vi "PRI.vi"(8 "Stopp":bool, 10 "SLOT":i32=100 min=0 max=999 step=100 format="%03d", 11 "USB":i32) -> ()   [LabVIEW 2020]
doc: "This VI provides a GUI for PRI modules. It implements an abstract module interface, where callers provide the only necessary and sufficient information for callee modules via the datafields USB, SLOT and Stopp. All module intern information are handled hidden by the module. Thereby, a caller must not \"know\" about such internals."
panel:
  out "Zeroed Intens":sgl[](array[numeric]) format="%.1f %%"
  in  "WL_Index":i32(ring) caption="Wavelength" items=["450 nm", "515 nm", "640 nm"]
  out "Wavelengths":i32[](array[numeric]) format="%.0f nm"
  in  "ZeroBtn":bool caption="Boolean"
  in  "Intensity":sgl min=0 max=100 step=1 format="%.1f %%"
  out "OnTime":i32=421 min=1000 max=200000000 step=1000 format="%5d ns"
  out "OffFactLo":i32=421 min=1000 max=200000000 step=1000 format="%5d * On-Time"
  out "OffFactHi":i32=421 min=1000 max=200000000 step=1000 format="%5d * On-Time"
  out "OnTimeLo":i32=421 min=1000 max=200000000 step=1000 format="%5d ns"
  out "OnTimeHi":i32=421 min=1000 max=200000000 step=1000 format="%5d ns"
  out "FreqLo":i32=421 min=1000 max=200000000 step=1000 format="%5d Hz"
  out "FreqHi":i32=421 min=1000 max=200000000 step=1000 format="%5d Hz"
  in  "FreqUnitPrefix":i32(ring) items=["Hz"=0, "kHz"=3, "MHz"=6]
  in  "Gating":enum32{"Timing", "Impedance"}(tab)
  in  "Gate Enabled":bool
  in  "OnTimeUnitPrefix":i32(ring) items=["s"=9, "ms"=6, "µs"=3, "ns"=0]
  in  "OnTimeMant":sgl=384.0 caption="On-Time" min=0 max=1000 step=1 format="%.1f"
  in  "OffFact":i32=255 caption="Off-Time" min=1 max=255 step=1 format="%5d * On-Time"
  in  "Gate Impedance":enum32{"   Low", "   High"}(radio)
  out "Frequency":i32=421 min=1000 max=200000000 step=1000 format="%5d Hz"
  out "error out":errorcluster caption="Error OUT"
  in  "FreqMant":sgl=384.0 caption="Frequency" min=0 max=1000 step=1
  out "NeedsFrequency":bool[](array[boolean])
  in  "Oper. Mode":i32(ring) items=["Off         ", "Narrow Pulse", "Broad Pulse ", "CW          "]
  out "NeedsTrigLvl":bool[](array[boolean])
  in  "Trig. Source":i32(ring) items=["internal      ", "ext. (NIM)    ", "ext. (TTL)    ", "ext. (falling)", "ext. (rising) "]
  in  "Trig. Level":i32=421 min=-1000 max=1000 step=50 format="%5d mV"
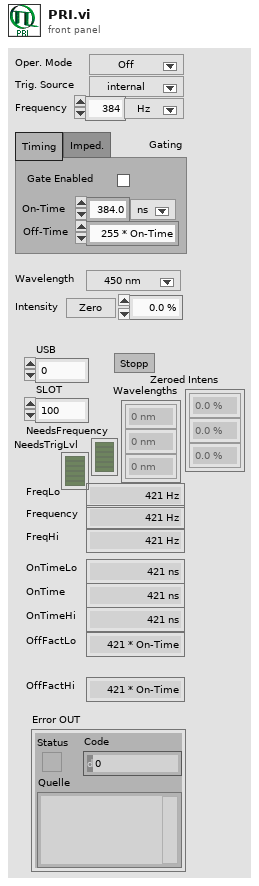
[diagram p1: front panel]
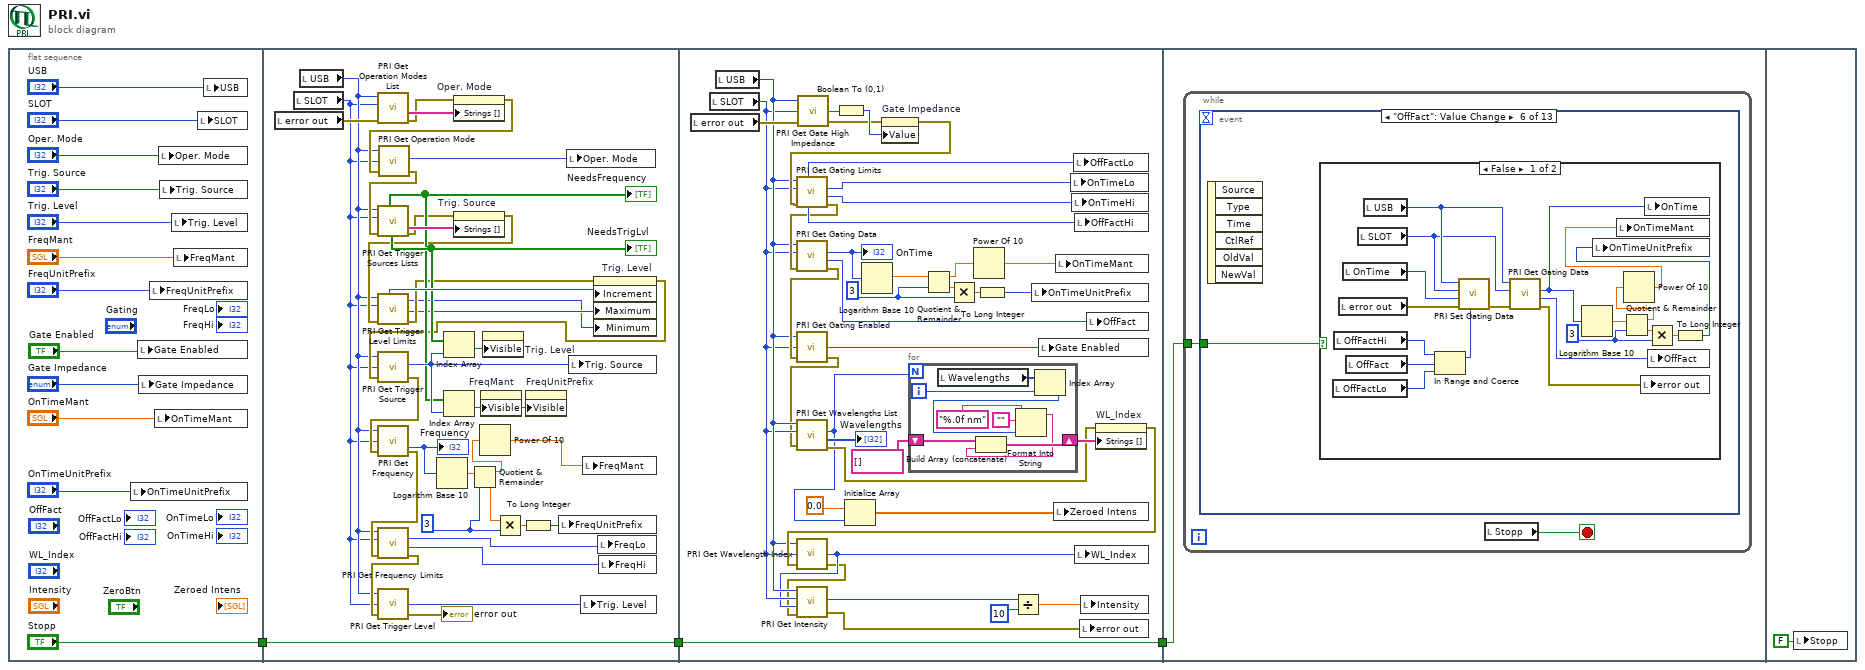
[diagram p0: block diagram]
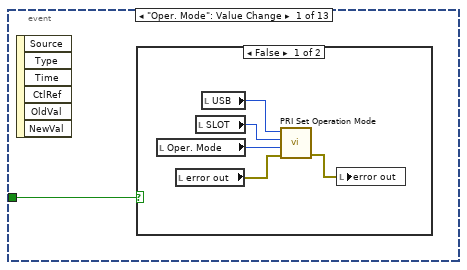
[diagram p2: hidden frame]
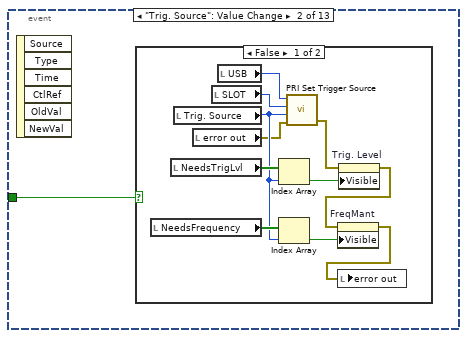
[diagram p4: hidden frame]
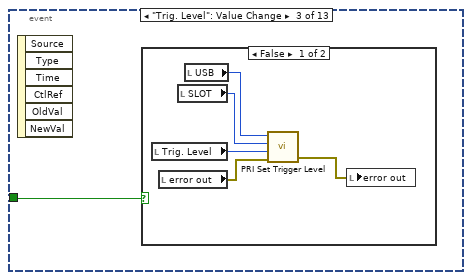
[diagram p6: hidden frame]
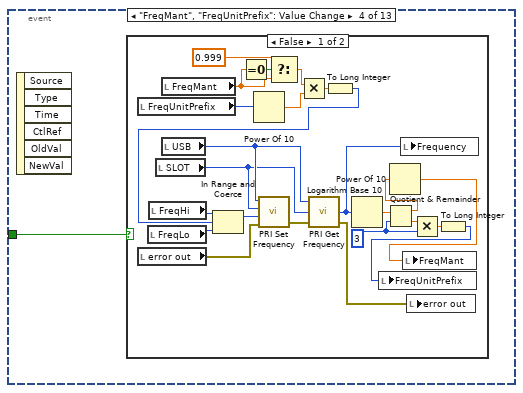
[diagram p8: hidden frame]
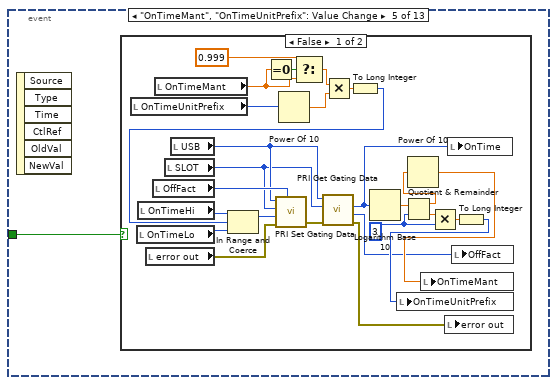
[diagram p10: hidden frame]
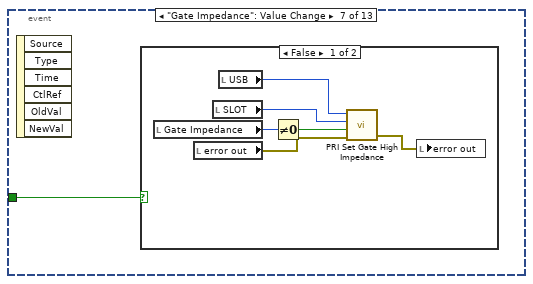
[diagram p13: hidden frame]
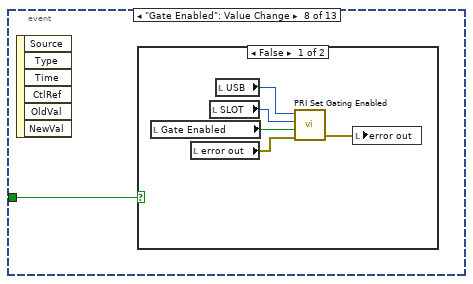
[diagram p15: hidden frame]
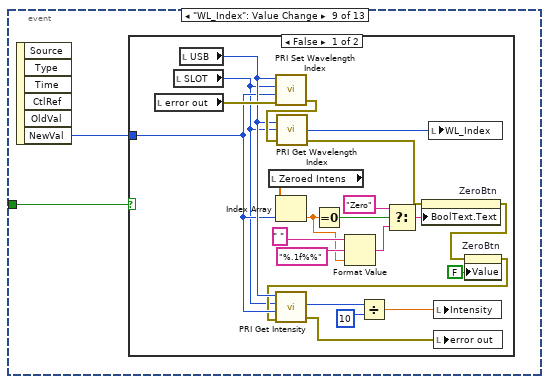
[diagram p17: hidden frame]
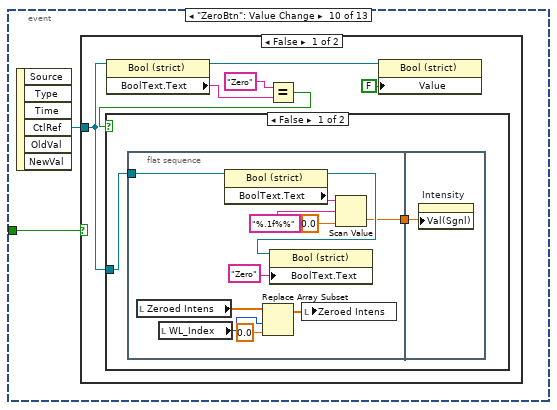
[diagram p19: hidden frame]
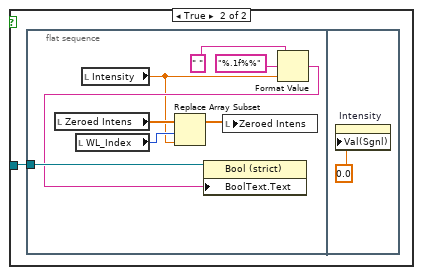
[diagram p20: hidden frame]
diagram:
  n1 = flat-sequence {
    tunnel: ["Stopp"] -> w3
    tunnel: [w51] -> w2
    tunnel: w3 -> [w51]
    tunnel: w2 -> [w91]
    tunnel: [w91] -> w1
    tunnel: w1 -> [w100]
    frame #0 {
      n2 = local write "OnTimeUnitPrefix"("OnTimeUnitPrefix") -> ()
      n3 = local write "Gate Enabled"("Gate Enabled") -> ()
      n4 = local write "Gate Impedance"("Gate Impedance") -> ()
      n5 = local write "FreqUnitPrefix"("FreqUnitPrefix") -> ()
      n6 = local write "OnTimeMant"("OnTimeMant") -> ()
      n7 = local write "Oper. Mode"("Oper. Mode") -> ()
      n8 = local write "Trig. Source"("Trig. Source") -> ()
      n9 = local write "Trig. Level"("Trig. Level") -> ()
      n10 = local write "FreqMant"("FreqMant") -> ()
      n11 = local write "SLOT"("SLOT") -> ()
      n12 = local write "USB"("USB") -> ()
    }
    frame #1 {
      w37 = 3 ("Frequency")
      n13 = local read "error out"() -> (w42:errorcluster)
      n14 = local read "SLOT"() -> (w17:i32)
      n15 = local read "USB"() -> (w18:i32)
      n16 = call "PRI Get Operation Modes List.vi"("error in (no error)"=w42, "SlotId"=w17, "DevIdx"=w18) -> ("error out"=w27:errorcluster, "OpModes_List"=w46:string[])  [unwired: 1 in, 2 out]
      n17 = property on="Oper. Mode" class="Ring (strict)"(error in=w27, "Strings []"=w46) -> (error out=w20:errorcluster)  [unwired: 1 in, 1 out]
      n18 = call "PRI Get Operation Mode.vi"("error in (no error)"=w20, "SlotId"=w17, "DevIdx"=w18) -> ("error out"=w19:errorcluster, "OpMode_Idx"=w16:i32)  [unwired: 1 out]
      n19 = call "PRI Get Trigger Sources Lists.vi"("error in (no error)"=w19, "SlotId"=w17, "DevIdx"=w18) -> ("error out"=w26:errorcluster, "TrigSrcs_List"=w49:string[], "TrigLvlEna"=w48:bool[], "FreqEna"=w44:bool[])  [unwired: 1 in, 2 out]
      "NeedsTrigLvl" <- w48
      "NeedsFrequency" <- w44
      n20 = property on="Trig. Source" class="Ring (strict)"(error in=w26, "Strings []"=w49) -> (error out=w25:errorcluster)  [unwired: 1 in, 1 out]
      n21 = call "PRI Get Trigger Level Limits.vi"("error in (no error)"=w25, "SlotId"=w17, "DevIdx"=w18) -> ("error out"=w24:errorcluster, "MaxLevel"=w23:i32, "MinLevel"=w22:i32, "Resolution"=w50:i32)  [unwired: 1 in, 1 out]
      n22 = local write "Oper. Mode"(w16) -> ()
      n23 = property on="Trig. Level" class="DigNum (strict)"(error in=w24, "Increment"=w50, "Maximum"=w23, "Minimum"=w22) -> (error out=w21:errorcluster)  [unwired: 1 in, 1 out]
      n24 = call "PRI Get Trigger Source.vi"("error in (no error)"=w21, "SlotId"=w17, "DevIdx"=w18) -> ("error out"=w36:errorcluster, "TrigSrc_Idx"=w45:i32)  [unwired: 1 out]
      n25 = call "PRI Get Frequency.vi"("error in (no error)"=w36, "SlotId"=w17, "DevIdx"=w18) -> ("error out"=w31:errorcluster, "Frequency"=w40:i32)  [unwired: 1 out]
      "Frequency" <- w40
      n26 = call "PRI Get Frequency Limits.vi"("error in (no error)"=w31, "SlotId"=w17, "DevIdx"=w18) -> ("error out"=w30:errorcluster, "MaxFreq"=w29:i32, "MinFreq"=w28:i32)  [unwired: 1 in, 1 out]
      n27 = call "PRI Get Trigger Level.vi"("error in (no error)"=w30, "SlotId"=w17, "DevIdx"=w18) -> ("error out"=→"error out":errorcluster, "TriggerLevel"=w47:i32)  [unwired: 1 out]
      n28 = Logarithm Base 10(1:w40) -> (0:w38:dbl)
      n29 = Index Array(array=w48, index=w45) -> (element=w52:bool)
      n30 = Index Array(array=w44, index=w45) -> (element=w39:bool)
      n31 = Quotient & Remainder(x=w38, y=w37) -> (x-y*floor(x/y)=w35:dbl, floor(x/y)=w41:dbl)
      n32 = Power Of 10(x=w35) -> (10^x=w32:dbl)
      n33 = property on="FreqMant" class="DigNum (strict)"("Visible"=w39) -> ()  [unwired: 2 in, 2 out]
      n34 = property on="Trig. Level" class="DigNum (strict)"("Visible"=w52) -> ()  [unwired: 2 in, 2 out]
      n35 = Multiply(x=w41, y=w37) -> (x*y=w33:dbl)
      n36 = To Long Integer(number=w33) -> (32bit integer=w34:i32)
      n37 = property on="FreqUnitPrefix" class="Ring (strict)"("Visible"=w39) -> ()  [unwired: 2 in, 2 out]
      n38 = local write "FreqUnitPrefix"(w34) -> ()
      n39 = local write "Trig. Source"(w45) -> ()
      n40 = local write "Trig. Level"(w47) -> ()
      n41 = local write "FreqMant"(w32) -> ()
      n42 = local write "FreqLo"(w28) -> ()
      n43 = local write "FreqHi"(w29) -> ()
    }
    frame #2 {
      w70 = 3 ("Frequency")
      n44 = local read "error out"() -> (w90:errorcluster)
      n45 = local read "SLOT"() -> (w65:i32)
      n46 = local read "USB"() -> (w66:i32)
      n47 = call "PRI Get Gate High Impedance.vi"("error in (no error)"=w90, "SlotId"=w65, "DevIdx"=w66) -> ("error out"=w87:errorcluster, "Gate High Impedance"=w89:bool)  [unwired: 1 out]
      n48 = Boolean To (0,1)(Boolean=w89) -> (0, 1=w88:i16)
      n49 = property on="Gate Impedance" class="RadioBtnsControl (strict)"(error in=w87, "Value"=w88) -> (error out=w86:errorcluster)  [unwired: 1 in, 1 out]
      n50 = call "PRI Get Gating Limits.vi"("error in (no error)"=w86, "SlotId"=w65, "DevIdx"=w66) -> ("error out"=w80:errorcluster, "MaxOnTime"=w83:i32, "MinOnTime"=w81:i32, "MaxOffTimeFactor"=w82:i32, "MinOffTimeFactor"=w84:i32)  [unwired: 1 in, 1 out]
      n51 = call "PRI Get Gating Data.vi"("error in (no error)"=w80, "SlotId"=w65, "DevIdx"=w66) -> ("error out"=w79:errorcluster, "OffTimeFactor"=w71:i32, "OnTime"=w74:i32)  [unwired: 1 in, 1 out]
      "OnTime" <- w74
      n52 = call "PRI Get Gating Enabled.vi"("error in (no error)"=w79, "SlotId"=w65, "DevIdx"=w66) -> ("error out"=w57:errorcluster, "Gating Enabled"=w85:bool)  [unwired: 1 out]
      n53 = call "PRI Get Wavelengths List.vi"("error in (no error)"=w57, "SlotId"=w65, "DevIdx"=w66) -> ("error out"=w58:errorcluster, "Wavelengths"=→"Wavelengths":i32[], "ListLen"=w53:i32)  [unwired: 1 in, 1 out]
      n54 = Initialize Array(sgl 0.0, w53) -> (w61:sgl[])
      n55 = Logarithm Base 10(1:w74) -> (0:w77:dbl)
      n56 = for {
        N: w53 -> [_]
        shift-right: [w98] -> w59
        shift-left: string[] [] -> [w99]
        i -> [w93]
        n57 = local read "Wavelengths"() -> (w94:i32[])
        n58 = Index Array(array=w94, index=w93) -> (element=w95:i32)
        n59 = Format Into String(format string="%.0f nm", initial string="", w95) -> (resulting string=w96:string)  [unwired: 1 in, 1 out]
        n60 = Build Array (concatenate)(w99, w96) -> (w98:string[])
      }
      n61 = Quotient & Remainder(x=w77, y=w70) -> (x-y*floor(x/y)=w76:dbl, floor(x/y)=w78:dbl)
      n62 = Multiply(x=w78, y=w70) -> (x*y=w75:dbl)
      n63 = Power Of 10(x=w76) -> (10^x=w73:dbl)
      n64 = To Long Integer(number=w75) -> (32bit integer=w72:i32)
      n65 = local write "OnTimeUnitPrefix"(w72) -> ()
      n66 = local write "Gate Enabled"(w85) -> ()
      n67 = local write "Zeroed Intens"(w61) -> ()
      n68 = local write "OnTimeMant"(w73) -> ()
      n69 = local write "OnTimeLo"(w81) -> ()
      n70 = local write "OnTimeHi"(w83) -> ()
      n71 = local write "OffFactLo"(w84) -> ()
      n72 = local write "OffFactHi"(w82) -> ()
      n73 = local write "OffFact"(w71) -> ()
      n74 = property on="WL_Index" class="Ring (strict)"(error in=w58, "Strings []"=w59) -> (error out=w67:errorcluster)  [unwired: 1 in, 1 out]
      n75 = call "PRI Get Wavelength Index.vi"("error in (no error)"=w67, "SlotId"=w65, "DevIdx"=w66) -> ("error out"=w54:errorcluster, "Wavelength_Idx"=w55:i32)  [unwired: 1 out]
      n76 = call "PRI Get Intensity.vi"("error in (no error)"=w54, "Wavelength Idx"=w55, "SlotId"=w65, "DevIdx"=w66) -> ("error out"=w64:errorcluster, "Intensity"=w63:u16)  [unwired: 1 out]
      n77 = Divide(x=w63, y=u16 10) -> (x/y=w56:dbl)
      n78 = local write "WL_Index"(w55) -> ()
      n79 = local write "error out"(w64) -> ()
      n80 = local write "Intensity"(w56) -> ()
    }
    frame #3 {
      n81 = while {
        tunnel: w100 -> [w101]
        stop <- w102 stop-if-true
        n82 = event shown="[5] \"OffFact\": Value Change" {
          selector: _ -> [_ _ _ _ _ _ _ _ _ _ _ _ _]
          dyn-events: _ -> [_ _ _ _ _ _ _ _ _ _ _ _ _]
          timeout: _ -> [_ _ _ _ _ _ _ _ _ _ _ _ _]
          tunnel: w101 -> [w103 w109 w121 w127 w152 w179 w199 w206 w213 w237 w269 _ _]
          event "Oper. Mode": Value Change {
            n83 = event-data() -> ()  [unwired: 1 in, 6 out]
            n84 = case shown="False" w103 {
              frame False {
                n85 = local read "Oper. Mode"() -> (w108:i32)
                n86 = local read "error out"() -> (w105:errorcluster)
                n87 = local read "SLOT"() -> (w106:i32)
                n88 = local read "USB"() -> (w107:i32)
                n89 = call "PRI Set Operation Mode.vi"("error in (no error)"=w105, "OpMode_Idx"=w108, "SlotId"=w106, "DevIdx"=w107) -> ("error out"=w104:errorcluster)  [unwired: 1 in, 1 out]
                n90 = local write "error out"(w104) -> ()
              }
              frame True {
              }
            }
          }
          event "Trig. Source": Value Change {
            n91 = event-data() -> ()  [unwired: 1 in, 6 out]
            n92 = case shown="False" w109 {
              frame False {
                n93 = local read "NeedsFrequency"() -> (w116:bool[])
                n94 = local read "NeedsTrigLvl"() -> (w117:bool[])
                n95 = local read "Trig. Source"() -> (w115:i32)
                n96 = local read "error out"() -> (w113:errorcluster)
                n97 = local read "SLOT"() -> (w118:i32)
                n98 = local read "USB"() -> (w119:i32)
                n99 = Index Array(array=w117, index=w115) -> (element=w120:bool)
                n100 = Index Array(array=w116, index=w115) -> (element=w114:bool)
                n101 = call "PRI Set Trigger Source.vi"("error in (no error)"=w113, "TrigSrc_Idx"=w115, "SlotId"=w118, "DevIdx"=w119) -> ("error out"=w112:errorcluster)  [unwired: 1 in, 1 out]
                n102 = property on="Trig. Level" class="DigNum (strict)"(error in=w112, "Visible"=w120) -> (error out=w111:errorcluster)  [unwired: 1 in, 1 out]
                n103 = property on="FreqMant" class="DigNum (strict)"(error in=w111, "Visible"=w114) -> (error out=w110:errorcluster)  [unwired: 1 in, 1 out]
                n104 = local write "error out"(w110) -> ()
              }
              frame True {
              }
            }
          }
          event "Trig. Level": Value Change {
            n105 = event-data() -> ()  [unwired: 1 in, 6 out]
            n106 = case shown="False" w121 {
              frame False {
                n107 = local read "Trig. Level"() -> (w126:i32)
                n108 = local read "error out"() -> (w123:errorcluster)
                n109 = local read "SLOT"() -> (w124:i32)
                n110 = local read "USB"() -> (w125:i32)
                n111 = call "PRI Set Trigger Level.vi"("error in (no error)"=w123, "TriggerLevel"=w126, "SlotId"=w124, "DevIdx"=w125) -> ("error out"=w122:errorcluster)  [unwired: 1 in, 1 out]
                n112 = local write "error out"(w122) -> ()
              }
              frame True {
              }
            }
          }
          event "FreqMant", "FreqUnitPrefix": Value Change {
            n113 = event-data() -> ()  [unwired: 1 in, 6 out]
            n114 = case shown="False" w127 {
              frame False {
                w141 = 3 ("Frequency")
                n115 = local read "FreqUnitPrefix"() -> (w147:i32)
                n116 = local read "error out"() -> (w151:errorcluster)
                n117 = local read "FreqLo"() -> (w131:i32)
                n118 = local read "FreqHi"() -> (w132:i32)
                n119 = local read "SLOT"() -> (w148:i32)
                n120 = local read "FreqMant"() -> (w135:sgl)
                n121 = local read "USB"() -> (w149:i32)
                n122 = Equal To 0?(x=w135) -> (x = 0?=w136:bool)
                n123 = Power Of 10(x=w147) -> (10^x=w146:dbl)
                n124 = Select(t=0.999, s=w136, f=w135) -> (s? t:f=w133:dbl)
                n125 = Multiply(x=w133, y=w146) -> (x*y=w144:dbl)
                n126 = To Long Integer(number=w144) -> (32bit integer=w128:i32)
                n127 = In Range and Coerce(upper limit=w132, x=w128, lower limit=w131) -> (coerced(x)=w130:i32)  [unwired: 1 out]
                n128 = call "PRI Set Frequency.vi"("error in (no error)"=w151, "Frequency"=w130, "SlotId"=w148, "DevIdx"=w149) -> ("error out"=w150:errorcluster)  [unwired: 1 in, 1 out]
                n129 = call "PRI Get Frequency.vi"("error in (no error)"=w150, "SlotId"=w148, "DevIdx"=w149) -> ("error out"=w145:errorcluster, "Frequency"=w129:i32)  [unwired: 1 out]
                n130 = Logarithm Base 10(1:w129) -> (0:w142:dbl)
                n131 = Quotient & Remainder(x=w142, y=w141) -> (x-y*floor(x/y)=w140:dbl, floor(x/y)=w143:dbl)
                n132 = Power Of 10(x=w140) -> (10^x=w137:dbl)
                n133 = local write "Frequency"(w129) -> ()
                n134 = local write "FreqMant"(w137) -> ()
                n135 = local write "error out"(w145) -> ()
                n136 = Multiply(x=w143, y=w141) -> (x*y=w139:dbl)
                n137 = To Long Integer(number=w139) -> (32bit integer=w138:i32)
                n138 = local write "FreqUnitPrefix"(w138) -> ()
              }
              frame True {
              }
            }
          }
          event "OnTimeMant", "OnTimeUnitPrefix": Value Change {
            n139 = event-data() -> ()  [unwired: 1 in, 6 out]
            n140 = case shown="False" w152 {
              frame False {
                w173 = 3 ("Frequency")
                n141 = local read "OnTimeUnitPrefix"() -> (w178:i32)
                n142 = local read "OnTimeLo"() -> (w163:i32)
                n143 = local read "OnTimeHi"() -> (w164:i32)
                n144 = local read "error out"() -> (w155:errorcluster)
                n145 = local read "OffFact"() -> (w160:i32)
                n146 = local read "OnTimeMant"() -> (w167:sgl)
                n147 = local read "SLOT"() -> (w157:i32)
                n148 = local read "USB"() -> (w158:i32)
                n149 = Equal To 0?(x=w167) -> (x = 0?=w168:bool)
                n150 = Power Of 10(x=w178) -> (10^x=w177:dbl)
                n151 = Select(t=0.999, s=w168, f=w167) -> (s? t:f=w165:dbl)
                n152 = Multiply(x=w165, y=w177) -> (x*y=w176:dbl)
                n153 = To Long Integer(number=w176) -> (32bit integer=w162:i32)
                n154 = In Range and Coerce(upper limit=w164, x=w162, lower limit=w163) -> (coerced(x)=w161:i32)  [unwired: 1 out]
                n155 = call "PRI Set Gating Data.vi"("DevIdx"=w158, "SlotId"=w157, "OnTime"=w161, "error in (no error)"=w155, "OffTimeFactor"=w160) -> ("error out"=w159:errorcluster)  [unwired: 1 in, 1 out]
                n156 = call "PRI Get Gating Data.vi"("error in (no error)"=w159, "SlotId"=w157, "DevIdx"=w158) -> ("error out"=w156:errorcluster, "OffTimeFactor"=w153:i32, "OnTime"=w154:i32)  [unwired: 1 in, 1 out]
                n157 = Logarithm Base 10(1:w154) -> (0:w174:dbl)
                n158 = Quotient & Remainder(x=w174, y=w173) -> (x-y*floor(x/y)=w172:dbl, floor(x/y)=w175:dbl)
                n159 = Power Of 10(x=w172) -> (10^x=w169:dbl)
                n160 = local write "OnTimeMant"(w169) -> ()
                n161 = Multiply(x=w175, y=w173) -> (x*y=w171:dbl)
                n162 = local write "error out"(w156) -> ()
                n163 = local write "OnTime"(w154) -> ()
                n164 = local write "OffFact"(w153) -> ()
                n165 = To Long Integer(number=w171) -> (32bit integer=w170:i32)
                n166 = local write "OnTimeUnitPrefix"(w170) -> ()
              }
              frame True {
              }
            }
          }
          event "OffFact": Value Change {
            n167 = event-data() -> ()  [unwired: 1 in, 6 out]
            n168 = case shown="False" w179 {
              frame False {
                w185 = 3 ("Frequency")
                n169 = local read "OffFactLo"() -> (w194:i32)
                n170 = local read "OffFactHi"() -> (w195:i32)
                n171 = local read "error out"() -> (w196:errorcluster)
                n172 = local read "OnTime"() -> (w197:i32)
                n173 = local read "OffFact"() -> (w193:i32)
                n174 = local read "SLOT"() -> (w190:i32)
                n175 = local read "USB"() -> (w191:i32)
                n176 = In Range and Coerce(upper limit=w195, x=w193, lower limit=w194) -> (coerced(x)=w192:i32)  [unwired: 1 out]
                n177 = call "PRI Set Gating Data.vi"("DevIdx"=w191, "SlotId"=w190, "OnTime"=w197, "error in (no error)"=w196, "OffTimeFactor"=w192) -> ("error out"=w198:errorcluster)  [unwired: 1 in, 1 out]
                n178 = call "PRI Get Gating Data.vi"("error in (no error)"=w198, "SlotId"=w190, "DevIdx"=w191) -> ("error out"=w189:errorcluster, "OffTimeFactor"=w188:i32, "OnTime"=w182:i32)  [unwired: 1 in, 1 out]
                n179 = Logarithm Base 10(1:w182) -> (0:w186:dbl)
                n180 = Quotient & Remainder(x=w186, y=w185) -> (x-y*floor(x/y)=w184:dbl, floor(x/y)=w187:dbl)
                n181 = Power Of 10(x=w184) -> (10^x=w181:dbl)
                n182 = local write "OnTimeMant"(w181) -> ()
                n183 = local write "error out"(w189) -> ()
                n184 = local write "OnTime"(w182) -> ()
                n185 = Multiply(x=w187, y=w185) -> (x*y=w183:dbl)
                n186 = local write "OffFact"(w188) -> ()
                n187 = To Long Integer(number=w183) -> (32bit integer=w180:i32)
                n188 = local write "OnTimeUnitPrefix"(w180) -> ()
              }
              frame True {
              }
            }
          }
          event "Gate Impedance": Value Change {
            n189 = event-data() -> ()  [unwired: 1 in, 6 out]
            n190 = case shown="False" w199 {
              frame False {
                n191 = local read "Gate Impedance"() -> (w202:enum32{"   Low", "   High"})
                n192 = local read "error out"() -> (w201:errorcluster)
                n193 = local read "SLOT"() -> (w204:i32)
                n194 = local read "USB"() -> (w205:i32)
                n195 = Not Equal To 0?(x=w202) -> (x != 0?=w203:bool)
                n196 = call "PRI Set Gate High Impedance.vi"("error in (no error)"=w201, "Gate High Impedance"=w203, "SlotId"=w204, "DevIdx"=w205) -> ("error out"=w200:errorcluster)  [unwired: 1 in, 1 out]
                n197 = local write "error out"(w200) -> ()
              }
              frame True {
              }
            }
          }
          event "Gate Enabled": Value Change {
            n198 = event-data() -> ()  [unwired: 1 in, 6 out]
            n199 = case shown="False" w206 {
              frame False {
                n200 = local read "Gate Enabled"() -> (w209:bool)
                n201 = local read "error out"() -> (w207:errorcluster)
                n202 = local read "SLOT"() -> (w210:i32)
                n203 = local read "USB"() -> (w211:i32)
                n204 = call "PRI Set Gating Enabled.vi"("error in (no error)"=w207, "Gating Enabled"=w209, "SlotId"=w210, "DevIdx"=w211) -> ("error out"=w208:errorcluster)  [unwired: 1 in, 1 out]
                n205 = local write "error out"(w208) -> ()
              }
              frame True {
              }
            }
          }
          event "WL_Index": Value Change {
            n206 = event-data() -> ("NewVal"=w212:i32)  [unwired: 1 in, 5 out]
            n207 = case shown="False" w213 {
              tunnel: w212 -> [w228 _]
              frame False {
                n208 = local read "error out"() -> (w235:errorcluster)
                n209 = local read "SLOT"() -> (w215:i32)
                n210 = local read "USB"() -> (w230:i32)
                n211 = local read "Zeroed Intens"() -> (w227:sgl[])
                n212 = call "PRI Set Wavelength Index.vi"("error in (no error)"=w235, "Wavelength_Idx"=w228, "SlotId"=w215, "DevIdx"=w230) -> ("error out"=w231:errorcluster)  [unwired: 1 in, 1 out]
                n213 = Index Array(array=w227, index=w228) -> (element=w216:sgl)
                n214 = call "PRI Get Wavelength Index.vi"("error in (no error)"=w231, "SlotId"=w215, "DevIdx"=w230) -> ("error out"=w219:errorcluster, "Wavelength_Idx"=w229:i32)  [unwired: 1 out]
                n215 = Equal To 0?(x=w216) -> (x = 0?=w221:bool)
                n216 = Format Value(string ("")=" ", format string="%.1f%%", value (0)=w216) -> (output string=w222:string)
                n217 = Select(t="Zero", s=w221, f=w222) -> (s? t:f=w226:string)
                n218 = property on="ZeroBtn" class="Bool (strict)"(error in=w219, "BoolText.Text"=w226) -> (error out=w218:errorcluster)  [unwired: 1 in, 1 out]
                n219 = local write "WL_Index"(w229) -> ()
                n220 = property on="ZeroBtn" class="Bool (strict)"(error in=w218, "Value"=FALSE (".not. x?")) -> (error out=w217:errorcluster)  [unwired: 1 in, 1 out]
                n221 = call "PRI Get Intensity.vi"("error in (no error)"=w217, "Wavelength Idx"=w228, "SlotId"=w215, "DevIdx"=w230) -> ("error out"=w232:errorcluster, "Intensity"=w233:u16)  [unwired: 1 out]
                n222 = Divide(x=w233, y=u16 10) -> (x/y=w214:dbl)
                n223 = local write "Intensity"(w214) -> ()
                n224 = local write "error out"(w232) -> ()
              }
              frame True {
              }
            }
          }
          event "ZeroBtn": Value Change {
            n225 = event-data() -> ("CtlRef"=w236:refnum<vi>)  [unwired: 1 in, 5 out]
            n226 = case shown="False" w237 {
              tunnel: w236 -> [w241 _]
              frame False {
                n227 = property class="Bool (strict)"(reference=w241) -> (reference out=w240:refnum<vi>, "BoolText.Text"=w243:string)  [unwired: 1 in, 1 out]
                n228 = Equal?(x="Zero", y=w243) -> (x = y?=w239:bool)
                n229 = case shown="False" w239 {
                  tunnel: w241 -> [w245 w258]
                  frame False {
                    n230 = flat-sequence {
                      tunnel: w245 -> [w251]
                      tunnel: [w250] -> w244
                      tunnel: w244 -> [w257]
                      frame #0 {
                        n231 = local read "Zeroed Intens"() -> (w249:sgl[])
                        n232 = local read "WL_Index"() -> (w247:i32)
                        n233 = property class="Bool (strict)"(reference=w251) -> (reference out=w254:refnum<vi>, "BoolText.Text"=w256:string)  [unwired: 1 in, 1 out]
                        n234 = Replace Array Subset(array=w249, new element=sgl 0.0 ("new element/subarray"), index=w247) -> (w246:sgl[])
                        n235 = property class="Bool (strict)"(reference=w254, "BoolText.Text"="Zero" ("Boolean Text.Text")) -> ()  [unwired: 1 in, 2 out]
                        n236 = local write "Zeroed Intens"(w246) -> ()
                        n237 = Scan Value(string=w256, format string="%.1f%%", default (0 dbl)=0.0) -> (value=w250:dbl)  [unwired: 1 out]
                      }
                      frame #1 {
                        n238 = property on="Intensity" class="DigNum (strict)"("Val(Sgnl)"=w257) -> ()  [unwired: 2 in, 2 out]
                      }
                    }
                  }
                  frame True {
                    n239 = flat-sequence {
                      tunnel: w258 -> [w265]
                      frame #0 {
                        n240 = local read "Zeroed Intens"() -> (w262:sgl[])
                        n241 = local read "WL_Index"() -> (w261:i32)
                        n242 = local read "Intensity"() -> (w259:sgl)
                        n243 = Replace Array Subset(array=w262, new element=w259, index=w261) -> (w260:sgl[])
                        n244 = local write "Zeroed Intens"(w260) -> ()
                        n245 = Format Value(string ("")=" ", format string="%.1f%%", value (0)=w259) -> (output string=w263:string)
                        n246 = property class="Bool (strict)"(reference=w265, "BoolText.Text"=w263) -> ()  [unwired: 1 in, 2 out]
                      }
                      frame #1 {
                        n247 = property on="Intensity" class="DigNum (strict)"("Val(Sgnl)"=0.0) -> ()  [unwired: 2 in, 2 out]
                      }
                    }
                  }
                }
                n248 = property class="Bool (strict)"(reference=w240, "Value"=FALSE) -> ()  [unwired: 1 in, 2 out]
              }
              frame True {
              }
            }
          }
          event "Intensity": Value Change {
            n249 = event-data() -> ("NewVal"=w268:sgl)  [unwired: 1 in, 5 out]
            n250 = case shown="False" w269 {
              tunnel: w268 -> [w280 _]
              frame False {
                n251 = Multiply(x=w280, y=sgl 10.0) -> (x*y=w283:sgl)
                n252 = local read "WL_Index"() -> (w273:i32)
                n253 = local read "error out"() -> (w278:errorcluster)
                n254 = Round To Nearest(number=w283) -> (nearest integer value=w282:sgl)
                n255 = local read "SLOT"() -> (w274:i32)
                n256 = local read "USB"() -> (w275:i32)
                n257 = To Unsigned Word Integer(number=w282) -> (unsigned 16bit integer=w279:u16)
                n258 = call "PRI Set Intensity.vi"("DevIdx"=w275, "SlotId"=w274, "Wavelength Idx"=w273, "error in (no error)"=w278, "Intensity"=w279) -> ("error out"=w277:errorcluster)  [unwired: 1 in, 1 out]
                n259 = call "PRI Get Intensity.vi"("error in (no error)"=w277, "Wavelength Idx"=w273, "SlotId"=w274, "DevIdx"=w275) -> ("error out"=w276:errorcluster, "Intensity"=w271:u16)  [unwired: 1 out]
                n260 = Divide(x=w271, y=u16 10) -> (x/y=w270:dbl)
                n261 = local write "Intensity"(w270) -> ()
                n262 = local write "error out"(w276) -> ()
              }
              frame True {
              }
            }
          }
          event "Stopp": Value Change {
            n263 = event-data() -> ()  [unwired: 1 in, 6 out]
            n264 = property on="Stopp" class="Bool (strict)"("Val(Sgnl)"=TRUE ("Value (Signaling)")) -> ()  [unwired: 2 in, 2 out]
          }
          event Timeout {
            n265 = event-data() -> ()  [unwired: 1 in, 2 out]
          }
        }
        n266 = local read "Stopp"() -> (w102:bool)
      }
    }
    frame #4 {
      n267 = local write "Stopp"(FALSE ("Stopp")) -> ()
    }
  }
